vi "Pockels-Calculate ref frame acquisition time.vi"(11 "Variables":T1 {"Dwell time" format="%#_6f"; "Sample Clock Rate" format="%#_6f"}) -> (3 "Theoretical acquisition duration of ref frame (us)":dbl)   [LabVIEW 2020]
uses:
  Typedefs/Pockels mod gen variables cluster.ctl
  Typedefs/Imaging Protocols enum.ctl
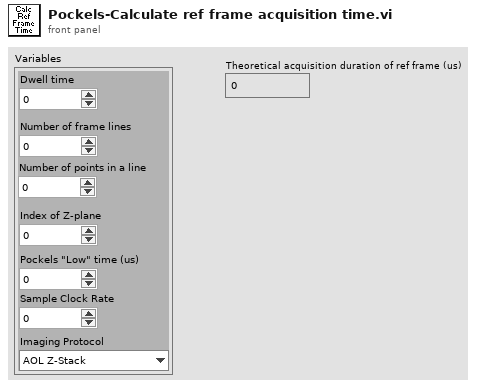
[diagram p1: front panel]
types:
  T1 = typedef "Pockels mod gen variables cluster.ctl" = cluster{"Dwell time":dbl, "Number of frame lines":i32, "Number of points in a line":i32, "Index of Z-plane":i32, "Pockels \"Low\" time (us)":dbl, "Sample Clock Rate":dbl, "Imaging Protocol":T2}
  T2 = typedef "Imaging Protocols enum.ctl" = enum16{"AOL Z-Stack", "Motor Z Stack", "Functional Acquisition", "Single Plane Acquisition", "Volume Acquisition", "Live Imaging", "Live Plane Imaging", "Live Volume Imaging"}
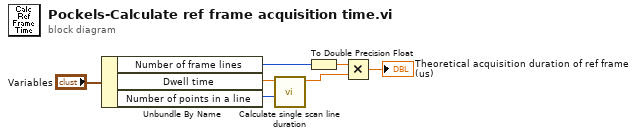
[diagram p0: block diagram]
diagram:
  n1 = Unbundle By Name("Variables") -> ("Number of frame lines"=w4:i32, "Dwell time"=w6:dbl, "Number of points in a line"=w5:i32)
  n2 = call "Calculate single scan line duration.vi"("Points in a scan line (~frame size)"=w5, "Dwell time (us)"=w6) -> ("Line scan time (us)"=w1:dbl)  [unwired: 9 in]
  n3 = To Double Precision Float(number=w4) -> (double precision float=w3:dbl)
  n4 = Multiply(x=w3, y=w1) -> (x*y=→"Theoretical acquisition duration of ref frame (us)":dbl)
